vi "Clear Index.vi"(8 "error in (no error)":errorcluster, 11 "Execution API In":refnum<class "Execution API.lvclass">) -> (0 "error out":errorcluster, 3 "Execution API Out":refnum<class "Execution API.lvclass">)   [LabVIEW 2020, in "Execution API.lvclass"]
doc: "Clear the index forcing it to be recreated when running tests."
uses:
  Execution API.lvclass
  Framework/Paths/Paths.lvlib
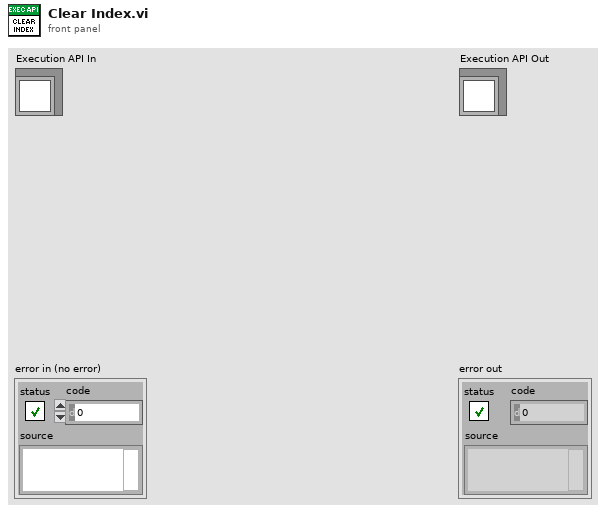
[diagram p1: front panel]
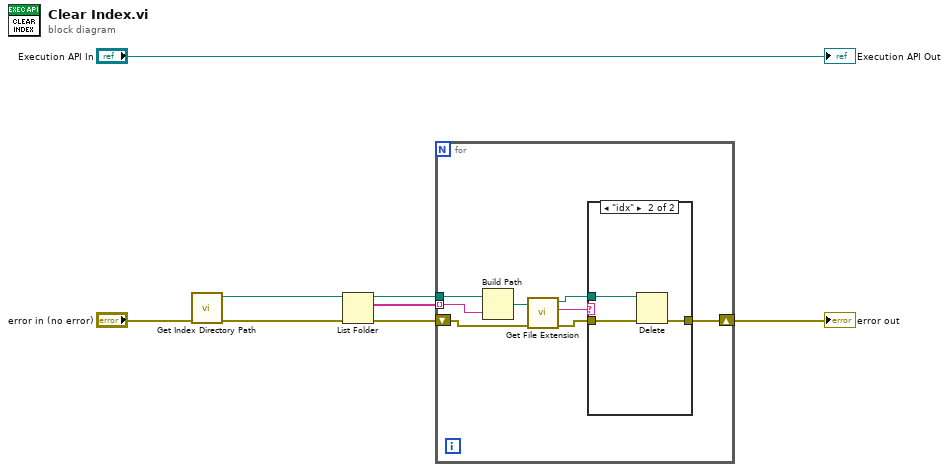
[diagram p0: block diagram]
diagram:
  n1 = call "Get Index Directory Path.vi"("error in (no error)"="error in (no error)") -> ("error out"=w2:errorcluster, "Index Directory"=w1:path)  [unwired: 9 in]
  n2 = List Folder(path=w1, error in=w2) -> (path out=w7:path, filenames=w6:string[], error out=w5:errorcluster)  [unwired: 2 in, 1 out]
  n3 = for {
    tunnel: w7 -> [w16]
    tunnel: w6 -> [w15] mode=indexing
    shift-right: [w13] -> w4
    shift-left: w5 -> [w14]
    n4 = Build Path(base path=w16, name or relative path=w15) -> (appended path=w11:path)
    n5 = call <vilib>:"Get File Extension.vi"("error in (no error)"=w14, "file"=w11) -> ("error out"=w12:errorcluster, "lowercase file extension"=w9:string, "dup file"=w10:path)  [unwired: 5 in, 2 out]
    n6 = case shown="\"idx\"" w9 {
      tunnel: [w17 w20] -> w13
      tunnel: w12 -> [w17 w19]
      tunnel: w10 -> [_ w18]
      frame Default {
      }
      frame "idx" {
        n7 = Delete(path (use dialog)=w18, error in=w19) -> (error out=w20:errorcluster)  [unwired: 3 in, 2 out]
      }
    }
  }
  "error out" <- w4
  "Execution API Out" <- "Execution API In"
